vi "Close_Relay.vi"() -> (5 "Plug in titles":string[](array[string]), 7 "Plug in values":string[](array[string]))   [LabVIEW 2016]
uses:
  Controls/Post_Process.ctl
  Globals/Meas_global.vi
panel:
  out "Current state":string
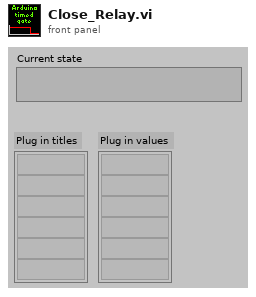
[diagram p1: front panel]
types:
  T1 = typedef "Post_Process.ctl" = enum16{"Take New Data", "Post Process Raw Data File"}
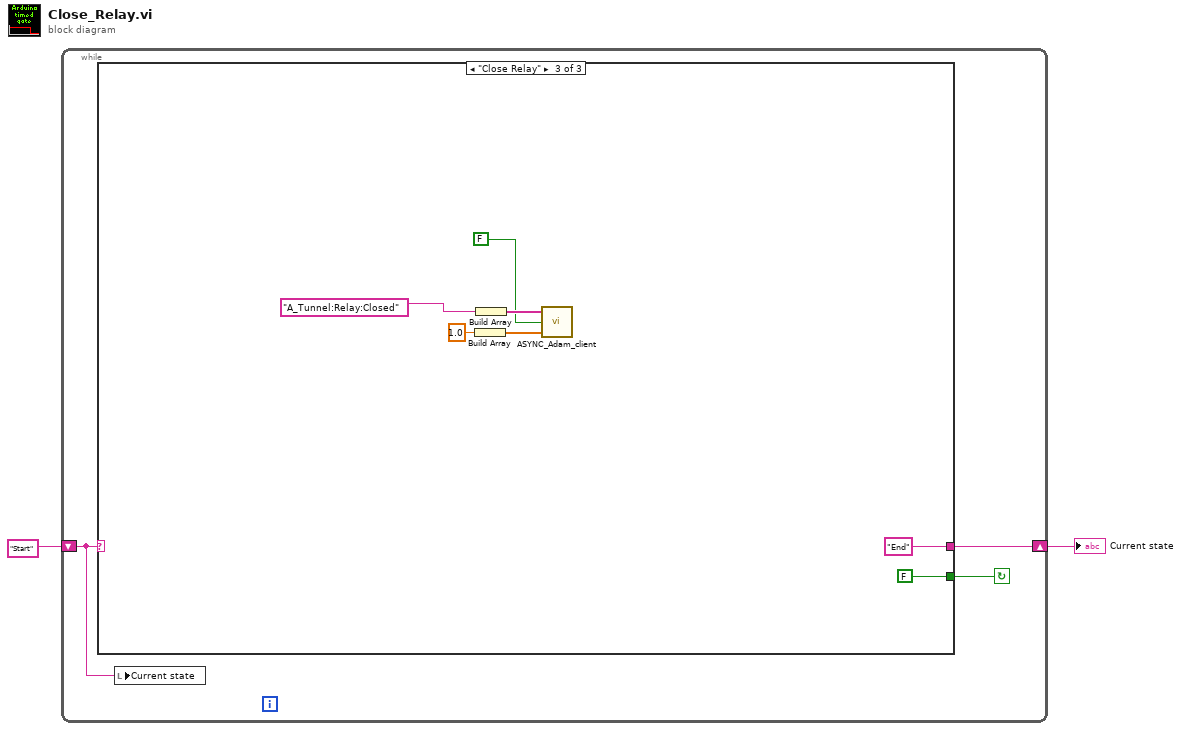
[diagram p0: block diagram]
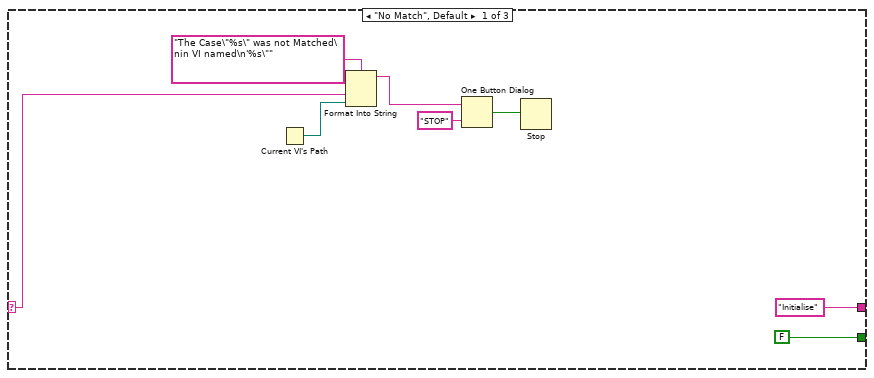
[diagram p2: hidden frame]
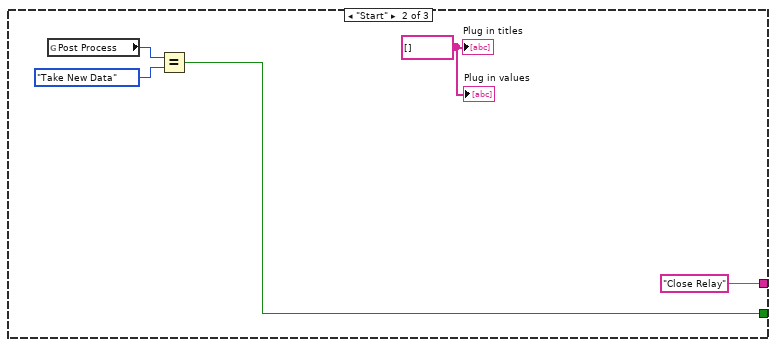
[diagram p3: hidden frame]
diagram:
  n1 = while {
    shift-left: "Start" -> [w3]
    shift-right: [w4] -> w1
    stop <- w5 continue-if-true
    n2 = case shown="\"Close Relay\"" w3 {
      selector: w3 -> [w6 _ _]
      tunnel: [FALSE w14 FALSE ("Command Found")] -> w5
      tunnel: ["Initialise" "Close Relay" "End"] -> w4
      frame "No Match", Default {
        n3 = Current VI's Path() -> (path=w8:path)
        n4 = Format Into String(format string="The Case\"%s\" was not Matched\nin VI named\n'%s\"" ("Format String"), w6, w8) -> (resulting string=w11:string)  [unwired: 2 in, 1 out]
        n5 = One Button Dialog(message=w11, button name ("OK")="STOP") -> (true=w9:bool)
        n6 = Stop(stop? (T)=w9) -> ()
      }
      frame "Start" {
        w15 = string[] [] ("Plug in titles")
        n7 = global read "Meas_global.vi" "Post Process"() -> (w16:T1)
        n8 = Equal?(x=w16, y=Post_Process."Take New Data" ("Post Process")) -> (x = y?=w14:bool)
        "Plug in values" <- w15
        "Plug in titles" <- w15
      }
      frame "Close Relay" {
        n9 = Build Array(1.0 ("element")) -> (w22:dbl[])
        n10 = Build Array("A_Tunnel:Relay:Closed") -> (w23:string[])
        n11 = call "ASYNC_Adam_client.vi"("Values"=w22, "Check Value is in the scan table?"=FALSE, "Channel Names"=w23) -> ()  [unwired: 2 out]
      }
    }
    n12 = local write "Current state"(w3) -> ()
  }
  "Current state" <- w1
